vi "Temp PalmSens.vi"() -> ()   [LabVIEW 2020]
uses:
  support/PCT FGV CMD.ctl
  <vilib>/regexp/Match Regular Expression.xnode
panel:
  out "whole match":string
  out "childs":string[][](array[string])
  in  "Text Ring":u16(ring) items=["Pretreatment settings (PS)", "Linear Sweep Voltammetry (LSV)", "Differential Pulse Voltammetry (DPV)", "Cyclic Voltammetry (CV)", "Chronoamperometry (CA)", "Chronopotentiometry (CP)", "El Imp Spectroscopy (EIS)"]
  in  "GET":bool
  out "NewVal":string
  in  "stop":bool
  in  "Tab Control":enum32{"Page 1", "Page 2"}(tab)
  in  "Tree":string(tree)
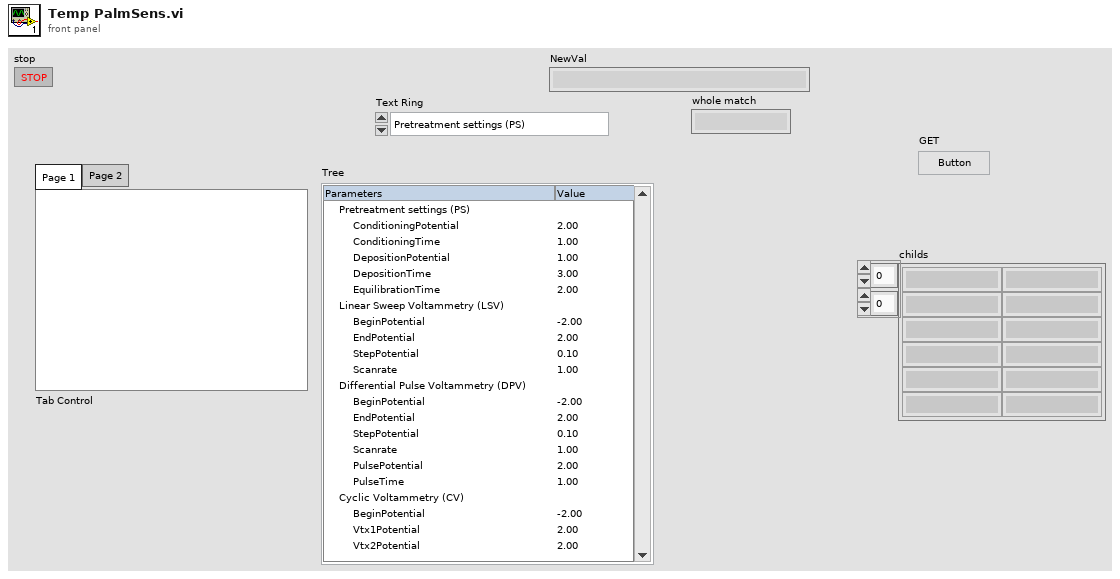
[diagram p1: front panel]
types:
  T1 = typedef "PCT FGV CMD.ctl" = enum16{"INIT", "GET", "SET"}
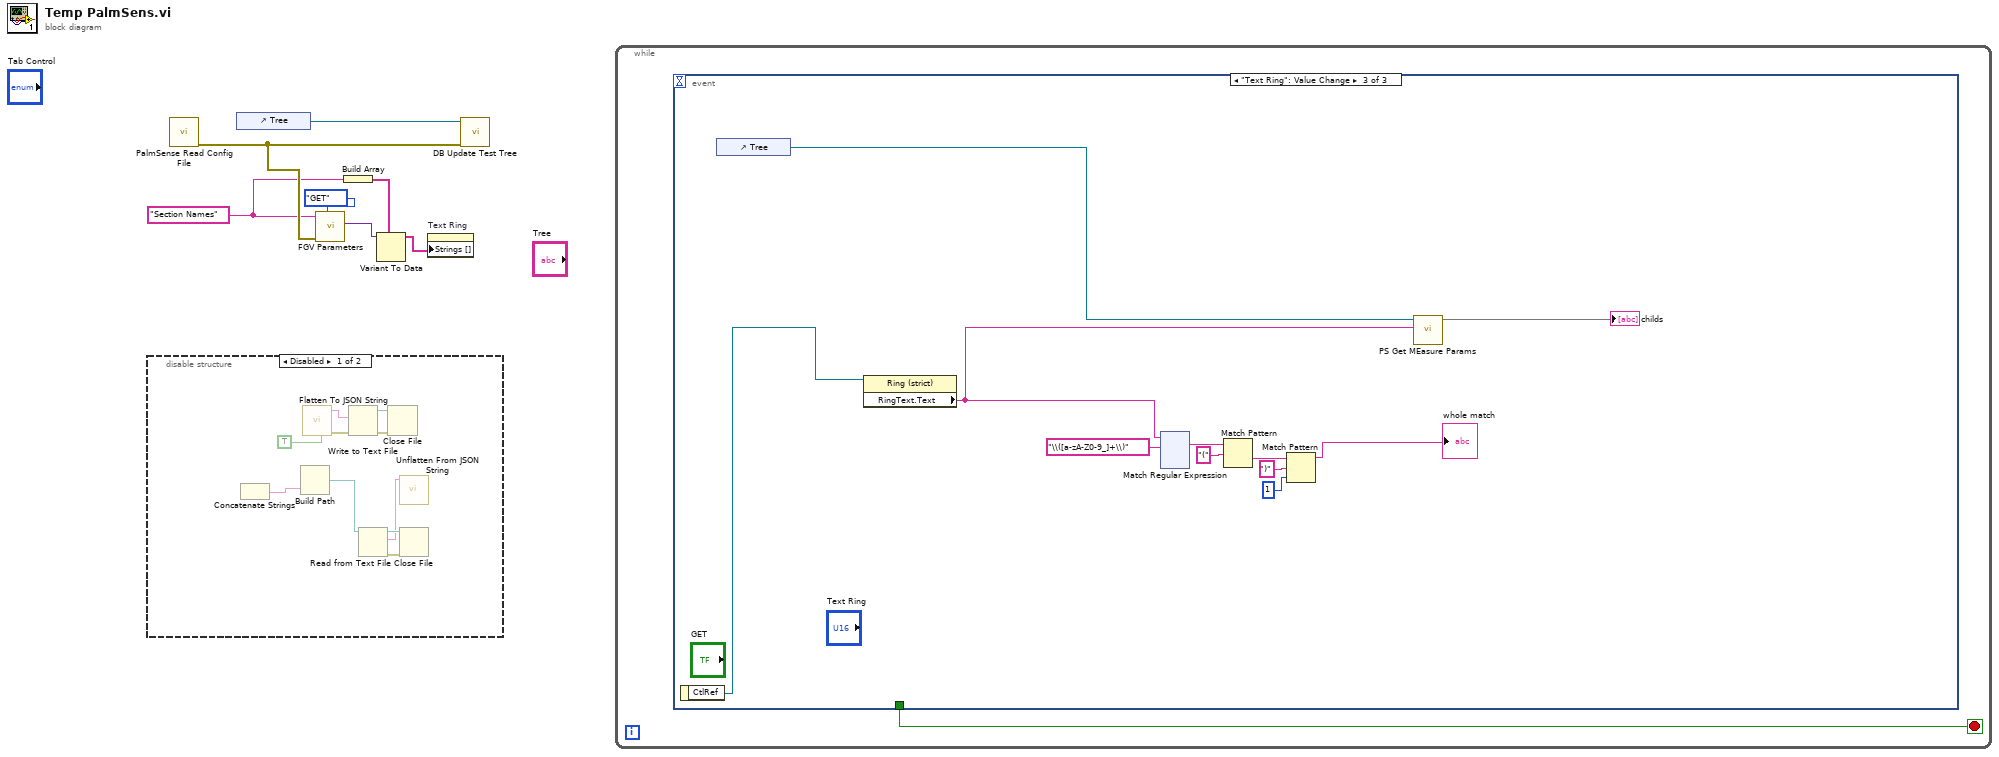
[diagram p0: block diagram]
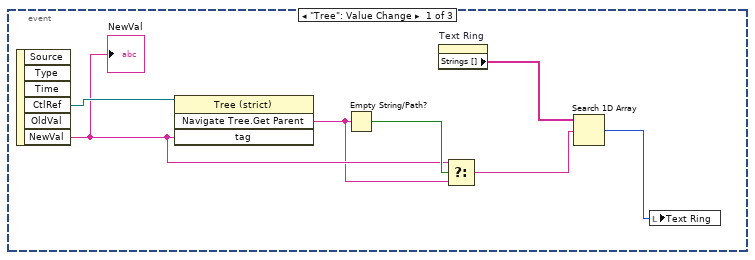
[diagram p3: hidden frame]
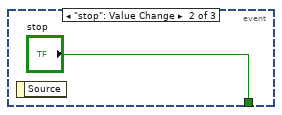
[diagram p4: hidden frame]
diagram:
  w3 = "Section Names"
  n1 = disable-structure shown="Disabled" {
    frame Disabled {
      n2 = Concatenate Strings() -> (w8:string)  [unwired: 2 in]
      n3 = Build Path(name or relative path=w8) -> (appended path=w12:path)  [unwired: 1 in]
      n4 = call <vilib>:"Flatten To JSON String.vi"("Enums As String (F)"=TRUE) -> ("error out"=w13:errorcluster, "JSON String"=w15:string)  [unwired: 9 in]
      n5 = Write to Text File(text=w15, error in=w13) -> (refnum out=w16:refnum<file>, error out=w17:errorcluster)  [unwired: 2 in, 1 out]
      n6 = Read from Text File(file (use dialog)=w12) -> (refnum out=w11:refnum<file>, text=w10:string, error out=w9:errorcluster)  [unwired: 3 in, 1 out]
      n7 = Close File(refnum=w16, error in=w17) -> ()  [unwired: 2 out]
      n8 = call <vilib>:"Unflatten From JSON String.vi"("JSON String"=w10) -> ()  [unwired: 9 in, 2 out]
      n9 = Close File(refnum=w11, error in=w9) -> ()  [unwired: 2 out]
    }
    frame Enabled {
    }
  }
  n10 = call "PalmSense Read Config File.vi"() -> ("error out"=w5:errorcluster)  [unwired: 11 in]
  n11 = control-ref of="Tree"() -> (w7:refnum<vi>)
  n12 = call "FGV Parameters.vi"("CMD"=PCT_FGV_CMD."GET", "error in (no error)"=w5, "Key"=w3) -> ("output"=w4:variant)  [unwired: 6 in, 2 out]
  n13 = Build Array(w3) -> (w2:string[])
  n14 = Variant To Data(type=w2, Variant=w4) -> (data=w1:string[])  [unwired: 1 in, 1 out]
  n15 = property on="Text Ring" class="Ring (strict)"("Strings []"=w1) -> ()  [unwired: 2 in, 2 out]
  n16 = call "DB Update Test Tree.vi"("error in (no error)"=w5, 11:w7) -> ()  [unwired: 9 in, 1 out]
  n17 = while {
    stop <- w18 stop-if-true
    n18 = event shown="[2] \"Text Ring\": Value Change" {
      selector: _ -> [_ _ _]
      dyn-events: _ -> [_ _ _]
      timeout: _ -> [_ _ _]
      tunnel: [_ "stop" _] -> w18
      event "Tree": Value Change {
        n19 = event-data() -> ("CtlRef"=w25:refnum<vi>, "NewVal"=w22:string)  [unwired: 1 in, 4 out]
        "NewVal" <- w22
        n20 = invoke class="Tree (strict)" method="Navigate Tree.Get Parent"(reference=w25, "tag"=w22) -> ("Navigate Tree:Get Parent"=w21:string)  [unwired: 2 in, 3 out]
        n21 = Empty String/Path?(string/path=w21) -> (empty?=w23:bool)
        n22 = property on="Text Ring" class="Ring (strict)"() -> ("Strings []"=w24:string[])  [unwired: 2 in, 2 out]
        n23 = Select(t=w22, s=w23, f=w21) -> (s? t:f=w20:string)
        n24 = Search 1D Array(1D array=w24, element=w20) -> (index of element=w19:i32)  [unwired: 1 in]
        n25 = local write "Text Ring"(w19) -> ()
      }
      event "stop": Value Change {
        n26 = event-data() -> ()  [unwired: 1 in, 1 out]
      }
      event "Text Ring": Value Change {
        n27 = event-data() -> ("CtlRef"=w35:refnum<vi>)  [unwired: 1 in]
        n28 = control-ref of="Tree"() -> (w37:refnum<vi>)
        n29 = property class="Ring (strict)"(reference=w35) -> ("RingText.Text"=w34:string)  [unwired: 1 in, 2 out]
        n30 = xnode "Match Regular Expression"("input string"=w34, "regular expression"="\\([a-zA-Z0-9_]+\\)") -> ("whole match"=w29:string)  [unwired: 4 in, 4 out]
        n31 = Match Pattern(string=w29, regular expression="(") -> (after substring=w27:string)  [unwired: 1 in, 3 out]
        n32 = Match Pattern(string=w27, regular expression=")", offset (0)=1) -> (before substring=→"whole match":string)  [unwired: 3 out]
        n33 = call "PS Get MEasure Params.vi"("Ring Text"=w34, "PS Measure Type 2"=w37) -> (3:→"childs")  [unwired: 9 in]
      }
    }
  }
